vi "simple_write_array.vi"(8 "error in (no error)":errorcluster, 9 "path":string, 10 "Array":dbl[](array[numeric]), 11 "hdf5_photon_record_log in":refnum<class "hdf5_photon_record_log.lvclass">) -> (0 "error out":errorcluster, 3 "hdf5_photon_record_log out":refnum<class "hdf5_photon_record_log.lvclass">)   [LabVIEW 2015, in "hdf5_photon_record_log.lvclass"]
uses:
  hdf5_photon_record_log.lvclass
  Data Logger Class/data_logger.lvclass
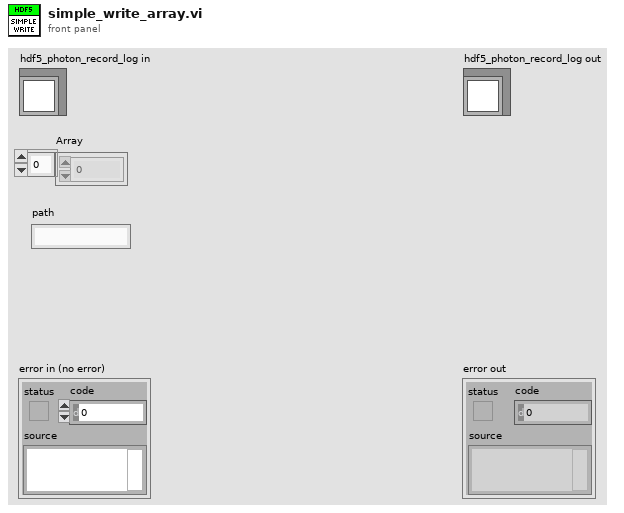
[diagram p1: front panel]
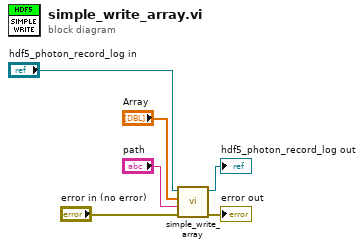
[diagram p0: block diagram]
diagram:
  n1 = call-parent "simple_write_array.vi"("error in (no error)"="error in (no error)", "path"="path", "Array"="Array", "data_logger in"="hdf5_photon_record_log in") -> ("error out"=→"error out":errorcluster, "data_logger out"=→"hdf5_photon_record_log out":refnum<class "hdf5_photon_record_log.lvclass">)  [unwired: 6 in]
